vi "Plugin FWLoader_A.vi"(4 "error in (no error)":errorcluster, 6 "Firmware file":path, 7 "Messaging Notifier":T1) -> (0 "error out":errorcluster, 1 "client ptr":i32, 2 "connection ptr":i32, 3 "Connected":bool)   [LabVIEW 2010, in "lib1299.lvlib"]
doc: "This VI loads the firmware into the DSP and restarts the DSP.\n\nInputs:\nStatus reference - reference to the status indicator used to display messages and status.\nFirmware file - firmware file to be loaded (*.bin)\nerror in - error input cluster\n\nOutputs:\nConnected - boolean indicator for connection status (TRUE = connected)\nconnection ptr - connection pointer for the estyx system\nclient ptr - client pointer for the estyx system\nerror out - error output cluster"
uses:
  lib1299.lvlib
  Controls/FW State.ctl
  Controls/TYP_Messaging Notifier Reference.ctl
panel:
  out "fw loader state":T2
  out "Status box":string
  out "Overall Progress":u8(slide) scale=0.0..7.0
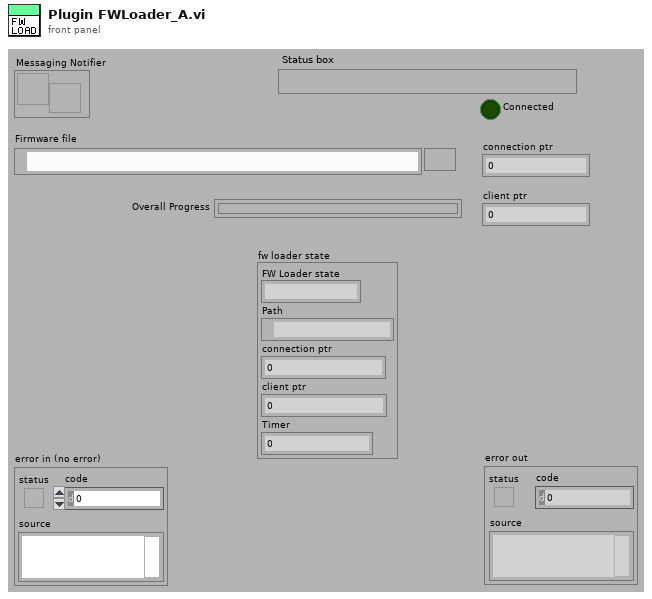
[diagram p1: front panel]
types:
  T1 = typedef "lib1299.lvlib/TYP_Messaging Notifier Reference.ctl" = refnum<notifier>
  T2 = typedef "lib1299.lvlib/FW State.ctl" = cluster{"FW Loader state":string, "Path":path, "connection ptr":i32, "client ptr":i32, "Timer":i64}
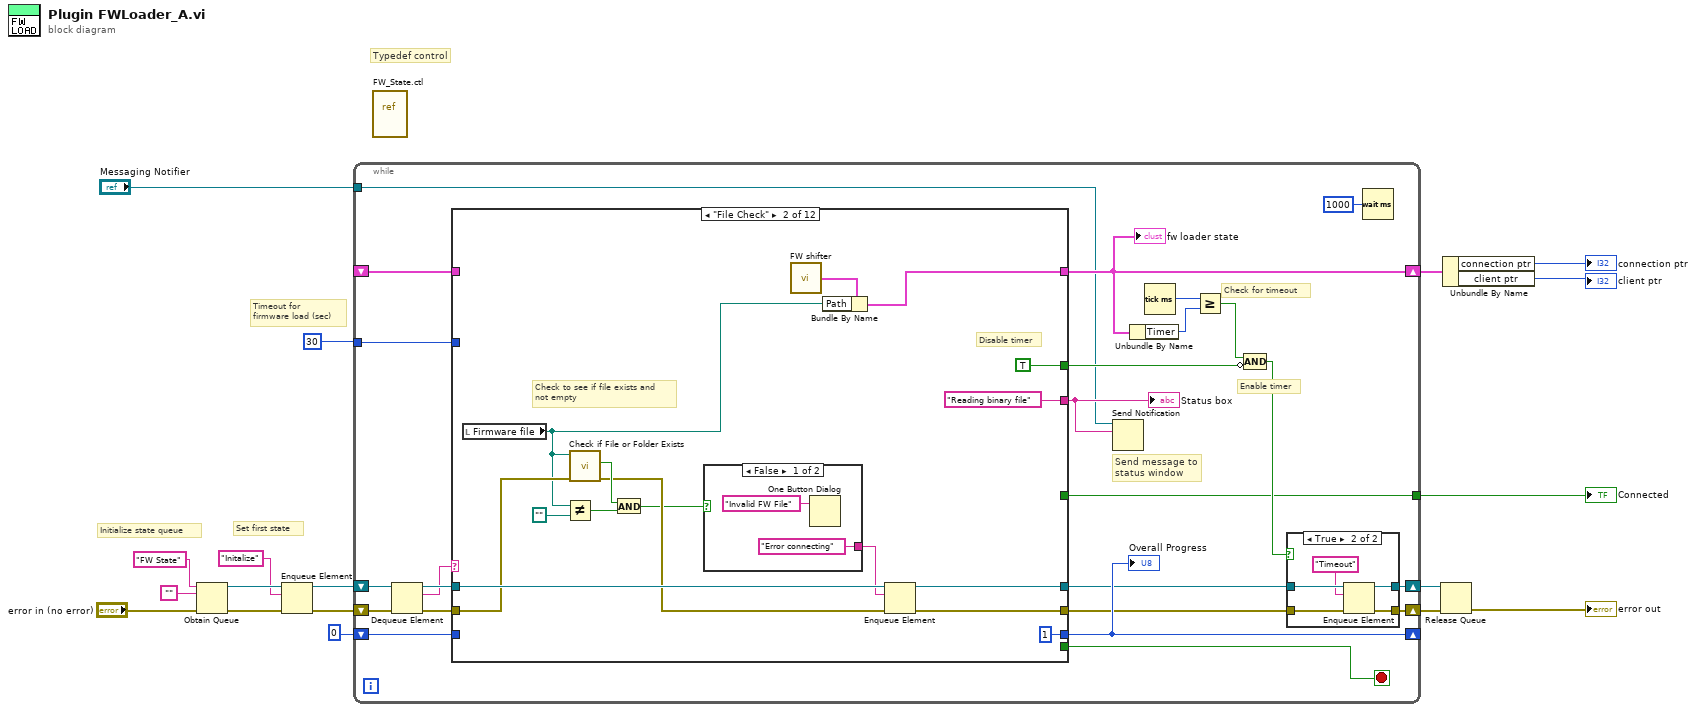
[diagram p0: block diagram]
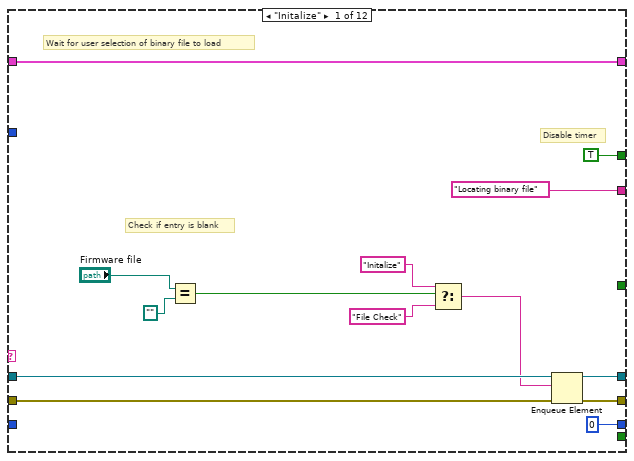
[diagram p3: hidden frame]
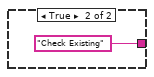
[diagram p4: hidden frame]
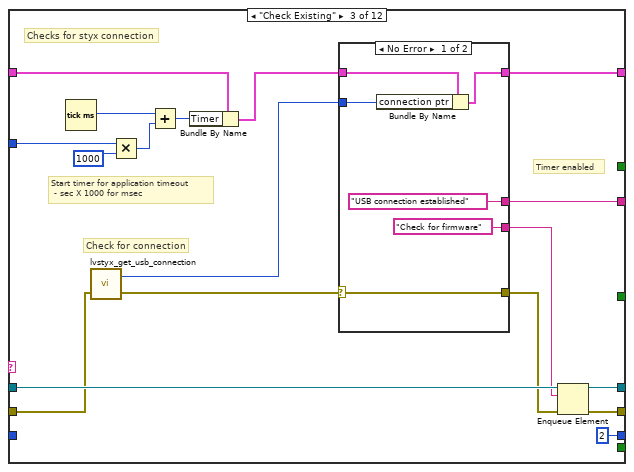
[diagram p5: hidden frame]
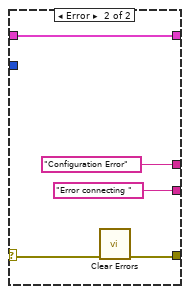
[diagram p6: hidden frame]
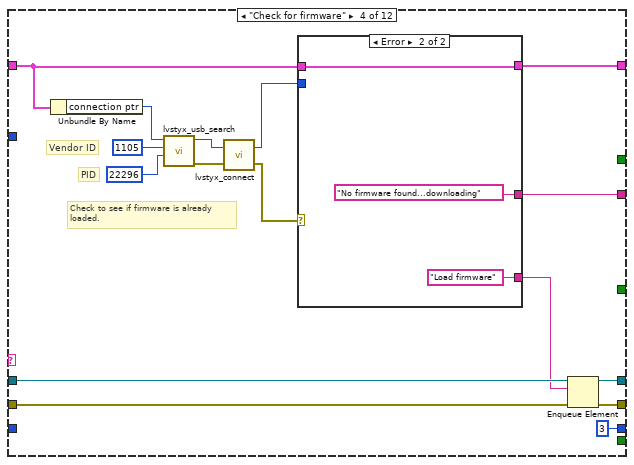
[diagram p7: hidden frame]
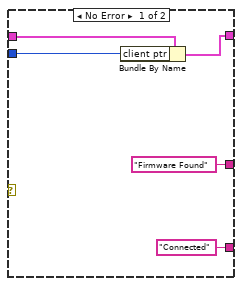
[diagram p8: hidden frame]
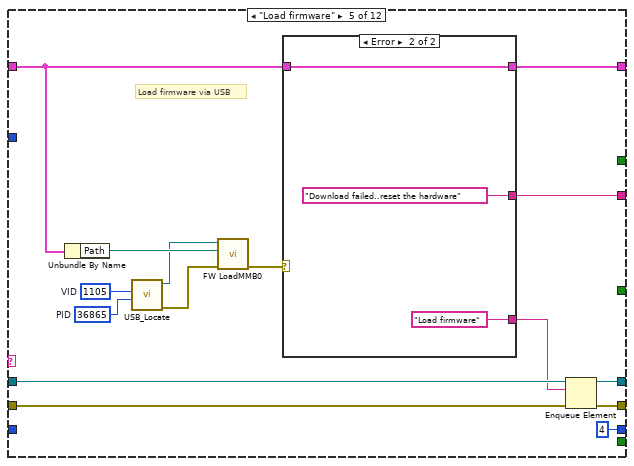
[diagram p9: hidden frame]
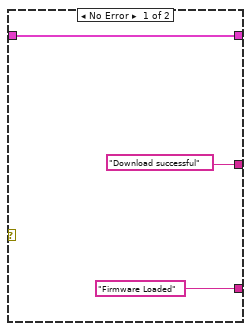
[diagram p10: hidden frame]
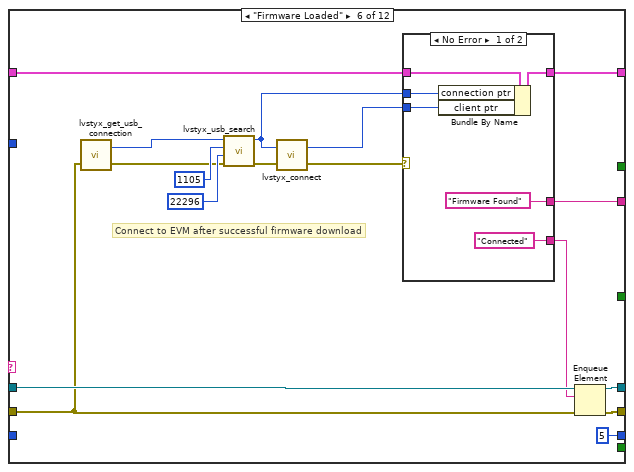
[diagram p11: hidden frame]
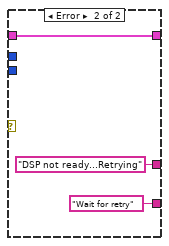
[diagram p12: hidden frame]
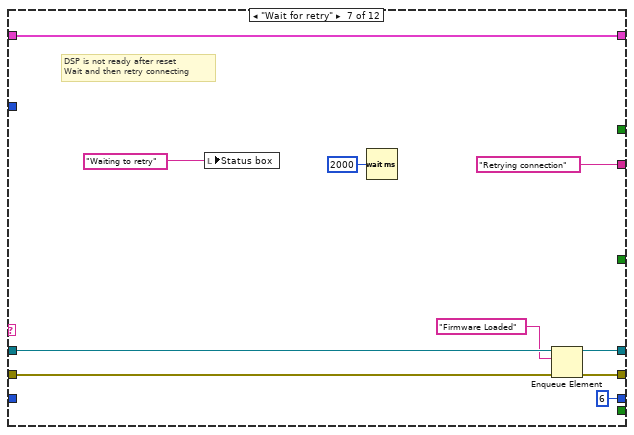
[diagram p13: hidden frame]
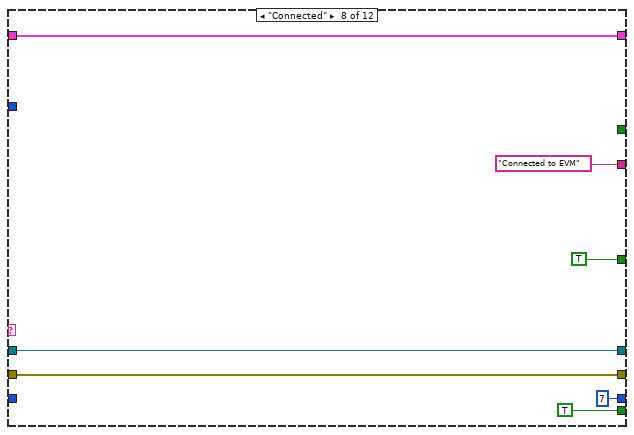
[diagram p14: hidden frame]
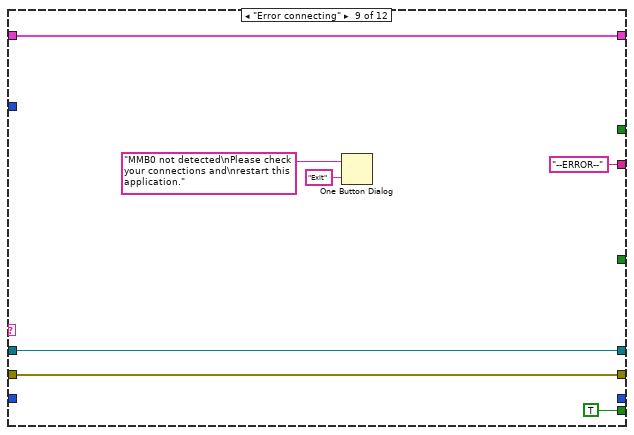
[diagram p15: hidden frame]
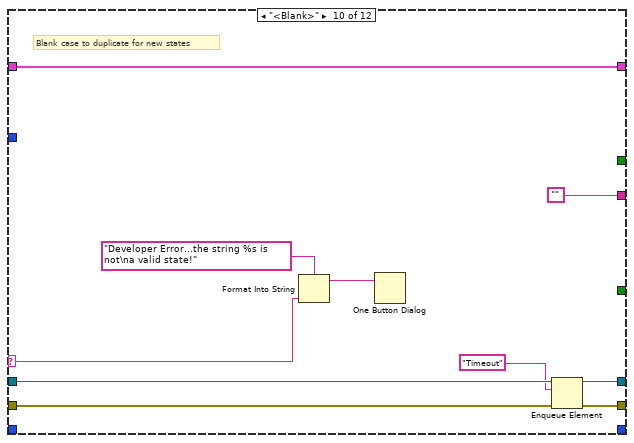
[diagram p16: hidden frame]
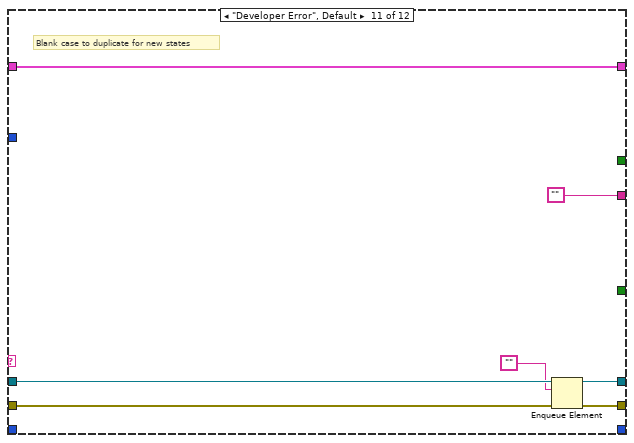
[diagram p17: hidden frame]
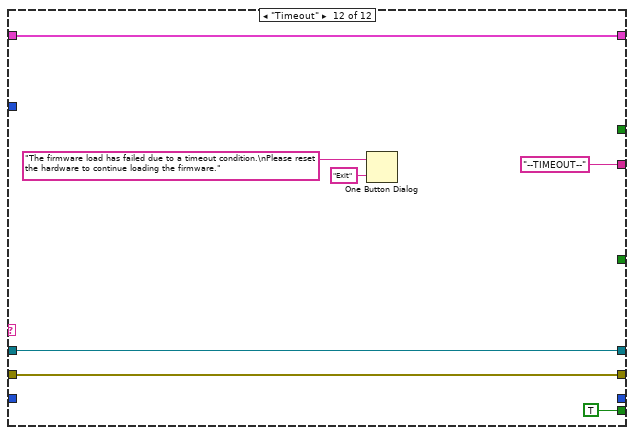
[diagram p18: hidden frame]
diagram:
  # "Typedef control"
  # "Set first state"
  # "Initialize state queue"
  # "Timeout for\nfirmware load (sec)"
  n1 = Obtain Queue(name (unnamed)="FW State", element data type="", error in (no error)="error in (no error)") -> (queue out=w18:refnum<queue>, error out=w17:errorcluster)  [unwired: 2 in, 1 out]
  n2 = Enqueue Element(queue=w18, element="Initalize", error in (no error)=w17) -> (queue out=w16:refnum<queue>, error out=w12:errorcluster)  [unwired: 1 in, 1 out]
  n3 = while {
    shift-right: [w35] -> w6
    shift-left: _ -> [w36]
    shift-right: [w23] -> w11
    shift-left: w12 -> [w37]
    shift-right: [w24] -> w10
    shift-left: w16 -> [w42]
    tunnel: 30 ("y") -> [w34]
    shift-right: [w28] -> _
    shift-left: 0 -> [w29]
    tunnel: [w21] -> w2
    tunnel: "Messaging Notifier" -> [w19]
    stop <- w27 stop-if-true
    # "Send message to \nstatus window"
    # "Enable timer"
    # "Check for timeout"
    n4 = Dequeue Element(queue=w42, error in (no error)=w37) -> (queue out=w41:refnum<queue>, element=w40:string, error out=w39:errorcluster)  [unwired: 1 in, 1 out]
    n5 = case shown="\"File Check\"" w40 {
      selector: w40 -> [_ _ _ _ _ _ _ _ _ w208 _ _]
      tunnel: w41 -> [w61 w76 w98 w125 w148 w171 w190 w199 w203 w214 w221 w229]
      tunnel: w39 -> [w60 w72 w97 w124 w147 w166 w189 w198 w202 w213 w220 w228]
      tunnel: [w63 w75 w100 w127 w150 w173 w192 w199 w203 w216 w223 w229] -> w26
      tunnel: [w59 w73 w93 w115 w142 w160 w188 w195 w206 w211 w217 w230] -> w35
      tunnel: [w62 w68 w99 w126 w149 w172 w191 w198 w202 w215 w222 w228] -> w25
      tunnel: w36 -> [w59 _ w86 w116 w141 w161 w188 w195 w206 w211 w217 w230]
      tunnel: ["Locating binary file" "Reading binary file" w91 w112 w144 w159 "Retrying connection" "Connected to EVM" "--ERROR--" "" "" "--TIMEOUT--"] -> w20
      tunnel: [_ _ _ _ _ _ _ TRUE TRUE _ _ TRUE] -> w27
      tunnel: w34 -> [_ _ w87 _ _ _ _ _ _ _ _ _]
      tunnel: [TRUE TRUE _ _ _ _ _ _ _ _ _ _] -> w31
      tunnel: w29 -> [_ _ _ _ _ _ _ _ _ _ _ _]
      tunnel: [0 1 2 3 4 5 6 7 _ _ _ _] -> w28
      tunnel: [_ _ _ _ _ _ _ TRUE _ _ _ _] -> w21
      frame "Initalize" {
        # "Disable timer"
        # "Check if entry is blank"
        # "Wait for user selection of binary file to load"
        n6 = Equal?(x="Firmware file", y=path "") -> (x = y?=w53:bool)
        n7 = Select(t="Initalize", s=w53, f="File Check") -> (s? t:f=w55:string)
        n8 = Enqueue Element(queue=w61, element=w55, error in (no error)=w60) -> (queue out=w63:refnum<queue>, error out=w62:errorcluster)  [unwired: 1 in, 1 out]
      }
      frame "File Check" {
        # "Check to see if file exists and\nnot empty"
        # "Disable timer"
        n9 = local read "Firmware file"() -> (w65:path)
        n10 = Not Equal?(x=w65, y=path "") -> (x != y?=w79:bool)
        n11 = call <vilib>:"Check if File or Folder Exists.vi"("error in (no error)"=w72, "path"=w65) -> ("error out"=w71:errorcluster, "file or folder exists?"=w78:bool)  [unwired: 7 in, 1 out]
        n12 = And(x=w78, y=w79) -> (x .and. y?=w70:bool)
        n13 = case shown="False" w70 {
          tunnel: ["Error connecting" "Check Existing"] -> w69
          frame False {
            n14 = One Button Dialog(message="Invalid FW File") -> ()  [unwired: 1 in, 1 out]
          }
          frame True {
          }
        }
        n15 = call "FW shifter.vi"() -> ("Cluster"=w74:T2)  [unwired: 1 in]
        n16 = Bundle By Name(cluster=w74, "Path"=w65) -> (w73:T2)
        n17 = Enqueue Element(queue=w76, element=w69, error in (no error)=w71) -> (queue out=w75:refnum<queue>, error out=w68:errorcluster)  [unwired: 1 in, 1 out]
      }
      frame "Check Existing" {
        # "Timer enabled"
        # "Checks for styx connection"
        # "Check for connection"
        # "Start timer for application timeout\n - sec X 1000 for msec"
        n18 = Tick Count (ms)() -> (millisecond timer value=w89:u32)
        n19 = call "lvstyx_get_usb_connection.vi"("error in (no error)"=w97) -> ("error out"=w96:errorcluster, "connection ptr"=w92:u32)  [unwired: 1 in]
        n20 = Multiply(x=w87, y=1000) -> (x*y=w90:i32)
        n21 = Add(x=w89, y=w90) -> (x+y=w84:u32)
        n22 = Bundle By Name(cluster=w86, "Timer"=w84) -> (w85:T2)
        n23 = case shown="No Error" w96 {
          selector: w96 -> [w106 w110]
          tunnel: [w106 w111] -> w95
          tunnel: ["Check for firmware" "Error connecting "] -> w94
          tunnel: w85 -> [w102 w107]
          tunnel: [w101 w107] -> w93
          tunnel: w92 -> [w103 _]
          tunnel: ["USB connection established" "Configuration Error"] -> w91
          frame No Error {
            n24 = Bundle By Name(cluster=w102, "connection ptr"=w103) -> (w101:T2)
          }
          frame Error {
            n25 = call <vilib>:"Clear Errors.vi"("error in (no error)"=w110) -> ("error out"=w111:errorcluster)  [unwired: 6 in]
          }
        }
        n26 = Enqueue Element(queue=w98, element=w94, error in (no error)=w95) -> (queue out=w100:refnum<queue>, error out=w99:errorcluster)  [unwired: 1 in, 1 out]
      }
      frame "Check for firmware" {
        # "PID"
        # "Vendor ID"
        # "Check to see if firmware is already\nloaded."
        n27 = Unbundle By Name(w116) -> ("connection ptr"=w120:i32)
        n28 = call "lvstyx_usb_search.vi"("pid"=u16 22296, "vid"=u16 1105, "conn ptr"=w120) -> ("error out"=w122:errorcluster, "dup conn ptr"=w118:u32)  [unwired: 6 in, 1 out]
        n29 = call "lvstyx_connect.vi"("error in (no error)"=w122, "connection ptr"=w118) -> ("error out"=w119:errorcluster, "client ptr"=w114:u32)
        n30 = case shown="Error" w119 {
          tunnel: ["Connected" "Load firmware"] -> w117
          tunnel: ["Firmware Found" "No firmware found...downloading"] -> w112
          tunnel: w116 -> [w130 w133]
          tunnel: [w129 w133] -> w115
          tunnel: w114 -> [w128 _]
          frame No Error {
            n31 = Bundle By Name(cluster=w130, "client ptr"=w128) -> (w129:T2)
          }
          frame Error {
          }
        }
        n32 = Enqueue Element(queue=w125, element=w117, error in (no error)=w124) -> (queue out=w127:refnum<queue>, error out=w126:errorcluster)  [unwired: 1 in, 1 out]
      }
      frame "Load firmware" {
        w136 = u16 36865  # PID
        w137 = u16 1105  # VID
        # "Load firmware via USB"
        n33 = Unbundle By Name(w141) -> ("Path"=w146:path)
        n34 = call "USB_Locate.vi"("pid"=w136, "vid"=w137) -> ("error out"=w139:errorcluster, "VISA Resource Name"=w138:refnum<visa-resource-name>)  [unwired: 7 in, 1 out]
        n35 = call "FW LoadMMB0.vi"("error in (no error)"=w139, "Boot file"=w146, "VISA resource name"=w138) -> ("error out"=w145:errorcluster)  [unwired: 8 in]
        n36 = case shown="Error" w145 {
          tunnel: ["Download successful" "Download failed..reset the hardware"] -> w144
          tunnel: ["Firmware Loaded" "Load firmware"] -> w143
          tunnel: [w151 w156] -> w142
          tunnel: w141 -> [w151 w156]
          frame No Error {
          }
          frame Error {
          }
        }
        n37 = Enqueue Element(queue=w148, element=w143, error in (no error)=w147) -> (queue out=w150:refnum<queue>, error out=w149:errorcluster)  [unwired: 1 in, 1 out]
      }
      frame "Firmware Loaded" {
        # "Connect to EVM after successful firmware download"
        n38 = call "lvstyx_get_usb_connection.vi"("error in (no error)"=w166) -> ("error out"=w165:errorcluster, "connection ptr"=w167:u32)  [unwired: 1 in]
        n39 = call "lvstyx_usb_search.vi"("error in (no error)"=w165, "pid"=u16 22296, "vid"=u16 1105, "conn ptr"=w167) -> ("error out"=w168:errorcluster, "dup conn ptr"=w162:u32)  [unwired: 5 in, 1 out]
        n40 = call "lvstyx_connect.vi"("error in (no error)"=w168, "connection ptr"=w162) -> ("error out"=w164:errorcluster, "client ptr"=w163:u32)
        n41 = case shown="No Error" w164 {
          tunnel: w163 -> [w176 _]
          tunnel: w162 -> [w177 _]
          tunnel: w161 -> [w179 w182]
          tunnel: [w178 w182] -> w160
          tunnel: ["Firmware Found" "DSP not ready...Retrying"] -> w159
          tunnel: ["Connected" "Wait for retry"] -> w158
          frame No Error {
            n42 = Bundle By Name(cluster=w179, "connection ptr"=w177, "client ptr"=w176) -> (w178:T2)
          }
          frame Error {
          }
        }
        n43 = Enqueue Element(queue=w171, element=w158, error in (no error)=w166) -> (queue out=w173:refnum<queue>, error out=w172:errorcluster)  [unwired: 1 in, 1 out]
      }
      frame "Wait for retry" {
        # "DSP is not ready after reset\nWait and then retry connecting"
        n44 = local write "Status box"("Waiting to retry") -> ()
        n45 = Wait (ms)(milliseconds to wait=u32 2000) -> ()  [unwired: 1 out]
        n46 = Enqueue Element(queue=w190, element="Firmware Loaded", error in (no error)=w189) -> (queue out=w192:refnum<queue>, error out=w191:errorcluster)  [unwired: 1 in, 1 out]
      }
      frame "Connected" {
      }
      frame "Error connecting" {
        n47 = One Button Dialog(message="MMB0 not detected\nPlease check your connections and\nrestart this application.", button name ("OK")="Exit") -> ()  [unwired: 1 out]
      }
      frame "<Blank>" {
        # "Blank case to duplicate for new states"
        n48 = Format Into String(format string="Developer Error...the string %s is not\na valid state!", w208) -> (resulting string=w209:string)  [unwired: 2 in, 1 out]
        n49 = One Button Dialog(message=w209) -> ()  [unwired: 1 in, 1 out]
        n50 = Enqueue Element(queue=w214, element="Timeout", error in (no error)=w213) -> (queue out=w216:refnum<queue>, error out=w215:errorcluster)  [unwired: 1 in, 1 out]
      }
      frame "Developer Error", Default {
        # "Blank case to duplicate for new states"
        n51 = Enqueue Element(queue=w221, element="", error in (no error)=w220) -> (queue out=w223:refnum<queue>, error out=w222:errorcluster)  [unwired: 1 in, 1 out]
      }
      frame "Timeout" {
        n52 = One Button Dialog(message="The firmware load has failed due to a timeout condition.\nPlease reset the hardware to continue loading the firmware.", button name ("OK")="Exit") -> ()  [unwired: 1 out]
      }
    }
    "fw loader state" <- w35
    "Status box" <- w20
    "Overall Progress" <- w28
    n53 = Send Notification(notification=w20, notifier=w19) -> ()  [unwired: 1 in, 2 out]
    n54 = Unbundle By Name(w35) -> ("Timer"=w32:i64)
    n55 = Tick Count (ms)() -> (millisecond timer value=w33:u32)
    n56 = Greater Or Equal?(x=w33, y=w32) -> (x >= y?=w30:bool)
    n57 = Compound Arithmetic op=AND(w30, invert w31) -> (w22:bool)
    n58 = case shown="True" w22 {
      tunnel: w26 -> [w44 w49]
      tunnel: w25 -> [w43 w48]
      tunnel: [w44 w47] -> w24
      tunnel: [w43 w46] -> w23
      frame False {
      }
      frame True {
        n59 = Enqueue Element(queue=w49, element="Timeout", error in (no error)=w48) -> (queue out=w47:refnum<queue>, error out=w46:errorcluster)  [unwired: 1 in, 1 out]
      }
    }
    n60 = Wait (ms)(milliseconds to wait=u32 1000) -> ()  [unwired: 1 out]
  }
  "Connected" <- w2
  n61 = vi-ref "FW_State.ctl"() -> ()  [unwired: 1 out]
  n62 = Release Queue(queue=w10, error in (no error)=w11) -> (error out=→"error out":errorcluster)  [unwired: 1 in, 2 out]
  n63 = Unbundle By Name(w6) -> ("connection ptr"=→"connection ptr":i32, "client ptr"=→"client ptr":i32)
